vi "PH_Periodic_Sequencer.panel.vi"() -> ()   [LabVIEW 2014, in "PH_Periodic_Sequencer.lvlib"]
uses:
  PH_Periodic_Sequencer.lvlib
  PH_StatusHandler/PH_StatusHandler.GUI element.ctl
  CSCore/CSSystem/CSSystemLib/CSSystemLib.lvlib
  PH_Common/PH_Common.lvlib
  PH_Class/PH_Class.lvlib
  PH_StatusHandler/PH_StatusHandler.lvlib
panel:
  out "Delivered Shots":i32
  in  "Wanted Shots":i32
  in  "Interval [sec]":dbl=-1.0
  out "FR":T1=2 caption="State PU"
  out "MA 5":T1=2 caption="State PU"
  out "MA 4":T1=2 caption="State PU"
  out "MA 3":T1=2 caption="State PU"
  out "MA 2":T1=2 caption="State PU"
  out "MA 1":T1=2 caption="State PU"
  out "45 DP":T1=2 caption="State PU"
  out "19 DP":T1=2 caption="State PU"
  out "Seq SM State":string="no info"
  out "Ready":u32(colorbox)
  in  "Start":bool
  in  "Main Off":bool
  out "error out":errorcluster
  in  "Delete":bool
  in  "error in (no error)":errorcluster
  in  "object ref":refnum<vi>
  # "PCS"
  # "3.40"
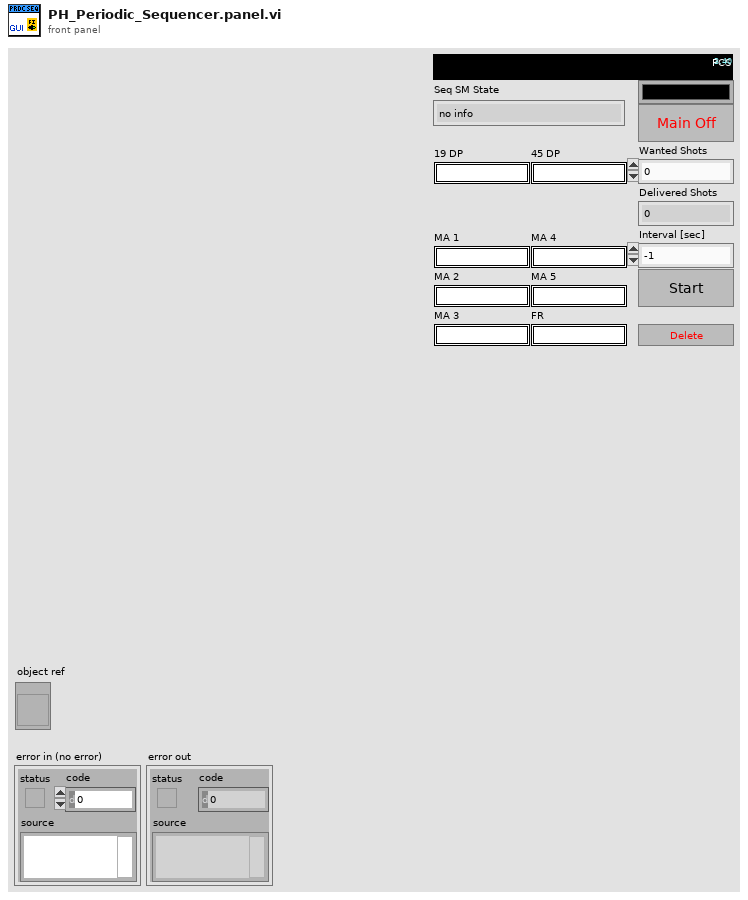
[diagram p1: front panel]
types:
  T1 = typedef "PH_StatusHandler.lvlib/PH_StatusHandler.GUI element.ctl" = u16
  T2 = typedef "PH_Periodic_Sequencer.lvlib/PH_Periodic_Sequencer.i attribute.ctl" = cluster{"GUI Refs":cluster{"Main Off":refnum<vi>, "Start":refnum<vi>, "Ready":refnum<vi>, "Sequencer SM State":refnum<vi>, "Interval [sec]":refnum<vi>, "Wanted Shots":refnum<vi>, "Delivered Shots":refnum<vi>}, "PU Info":cluster{"Instancename":string, "State":T3, "linked":bool}[], "Sequencer":cluster{"Instancename":string, "linked?":bool, "R2S?":bool, "SM State":string}, "Run?":bool, "Interval [sec]":dbl, "PU State Refs":refnum<vi>[], "Wanted Shots":i32, "Delivered Shots":i32}
  T3 = typedef "PH_StatusHandler.lvlib/PH_StatusHandler.Status.ctl" = i16
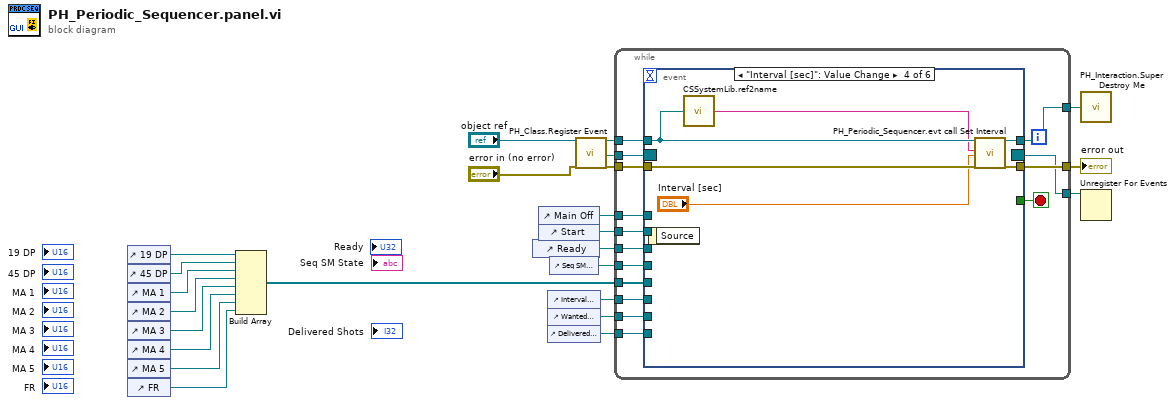
[diagram p0: block diagram]
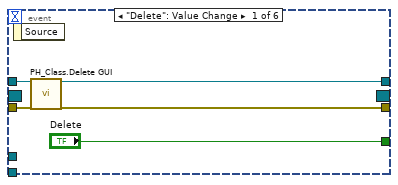
[diagram p2: hidden frame]
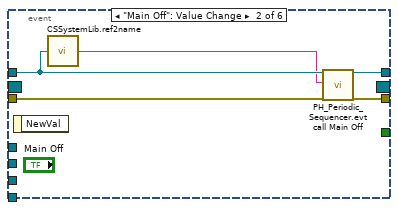
[diagram p3: hidden frame]
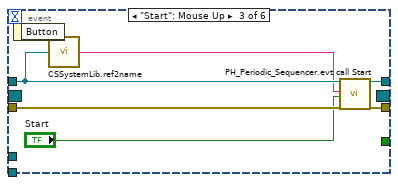
[diagram p4: hidden frame]
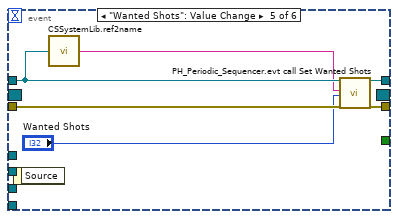
[diagram p5: hidden frame]
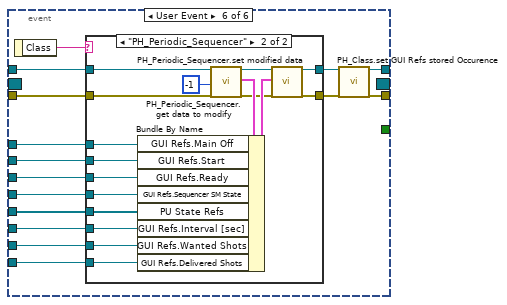
[diagram p6: hidden frame]
diagram:
  n1 = control-ref of="19 DP"() -> (w8:refnum<vi>)
  n2 = control-ref of="45 DP"() -> (w7:refnum<vi>)
  n3 = control-ref of="MA 1"() -> (w6:refnum<vi>)
  n4 = control-ref of="MA 2"() -> (w5:refnum<vi>)
  n5 = control-ref of="MA 3"() -> (w4:refnum<vi>)
  n6 = control-ref of="MA 4"() -> (w3:refnum<vi>)
  n7 = control-ref of="MA 5"() -> (w2:refnum<vi>)
  n8 = control-ref of="FR"() -> (w1:refnum<vi>)
  n9 = Build Array(w8, w7, w6, w5, w4, w3, w2, w1) -> (w14:refnum<vi>[])
  n10 = control-ref of="Ready"() -> (w16:refnum<vi>)
  n11 = control-ref of="Main Off"() -> (w18:refnum<vi>)
  n12 = control-ref of="Start"() -> (w17:refnum<vi>)
  n13 = control-ref of="Interval [sec]"() -> (w13:refnum<vi>)
  n14 = control-ref of="Wanted Shots"() -> (w12:refnum<vi>)
  n15 = control-ref of="Delivered Shots"() -> (w11:refnum<vi>)
  n16 = control-ref of="Seq SM State"() -> (w15:refnum<vi>)
  n17 = call "PH_Class.Register Event.vi"("i ref in"="object ref", "error in (no error)"="error in (no error)") -> ("i ref out"=w22:refnum<vi>, "Event Registration Refnum"=w20:refnum<event-registration>, "error out"=w21:errorcluster)  [unwired: 15 in]
  n18 = while {
    tunnel: w22 -> [w36]
    tunnel: [w35] -> w24
    tunnel: [w38] -> w23
    tunnel: w21 -> [w37]
    tunnel: w20 -> [w34]
    tunnel: [w33] -> w19
    tunnel: w18 -> [w32]
    tunnel: w17 -> [w31]
    tunnel: w16 -> [w30]
    tunnel: w15 -> [w29]
    tunnel: w14 -> [w28]
    tunnel: w13 -> [w27]
    tunnel: w12 -> [w26]
    tunnel: w11 -> [w25]
    stop <- w39 stop-if-true
    n19 = event shown="[3] \"Interval [sec]\": Value Change" {
      selector: w34 -> [_ _ _ _ _ _]
      dyn-events: [_ _ _ _ _ _] -> w33
      timeout: _ -> [_ _ _ _ _ _]
      tunnel: ["Delete" _ _ _ _ _] -> w39
      tunnel: w36 -> [w43 w47 w53 w59 w65 w80]
      tunnel: [w40 w48 w54 w60 w66 w81] -> w38
      tunnel: w37 -> [w42 w49 w55 w61 w67 w78]
      tunnel: [w41 w45 w51 w57 w63 w82] -> w35
      tunnel: w32 -> [_ _ _ _ _ w75]
      tunnel: w31 -> [_ _ _ _ _ w74]
      tunnel: w30 -> [_ _ _ _ _ w73]
      tunnel: w29 -> [_ _ _ _ _ w72]
      tunnel: w28 -> [_ _ _ _ _ w71]
      tunnel: w27 -> [_ _ _ _ _ w70]
      tunnel: w26 -> [_ _ _ _ _ w69]
      tunnel: w25 -> [_ _ _ _ _ w68]
      event "Delete": Value Change {
        n20 = event-data() -> ()  [unwired: 1 in, 1 out]
        n21 = call "PH_Class.Delete GUI.vi"("VI in"=w43, "error in (no error)"=w42) -> ("VI out"=w41:refnum<vi>, "error out"=w40:errorcluster)  [unwired: 16 in]
      }
      event "Main Off": Value Change {
        n22 = event-data() -> ()  [unwired: 1 in, 1 out]
        n23 = call "CSSystemLib.ref2name.vi"("obj refnum"=w47) -> ("name"=w46:string)
        n24 = call "PH_Periodic_Sequencer.evt call Main Off.vi"("i ref in"=w47, "Instance"=w46, "error in (no error)"=w49) -> ("i ref out"=w45:refnum<vi>, "error out"=w48:errorcluster)  [unwired: 15 in]
      }
      event "Start": Mouse Up {
        n25 = event-data() -> ()  [unwired: 1 in, 1 out]
        n26 = call "CSSystemLib.ref2name.vi"("obj refnum"=w53) -> ("name"=w52:string)
        n27 = call "PH_Periodic_Sequencer.evt call Start.vi"("i ref in"=w53, "Instance"=w52, "Start"="Start", "error in (no error)"=w55) -> ("i ref out"=w51:refnum<vi>, "error out"=w54:errorcluster)  [unwired: 14 in]
      }
      event "Interval [sec]": Value Change {
        n28 = event-data() -> ()  [unwired: 1 in, 1 out]
        n29 = call "CSSystemLib.ref2name.vi"("obj refnum"=w59) -> ("name"=w58:string)
        n30 = call "PH_Periodic_Sequencer.evt call Set Interval.vi"("i ref in"=w59, "Instance"=w58, "Interval [sec]"="Interval [sec]", "error in (no error)"=w61) -> ("i ref out"=w57:refnum<vi>, "error out"=w60:errorcluster)  [unwired: 14 in]
      }
      event "Wanted Shots": Value Change {
        n31 = event-data() -> ()  [unwired: 1 in, 1 out]
        n32 = call "CSSystemLib.ref2name.vi"("obj refnum"=w65) -> ("name"=w64:string)
        n33 = call "PH_Periodic_Sequencer.evt call Set Wanted Shots.vi"("i ref in"=w65, "Instance"=w64, "Wanted Shots"="Wanted Shots", "error in (no error)"=w67) -> ("i ref out"=w63:refnum<vi>, "error out"=w66:errorcluster)  [unwired: 14 in]
      }
      event User Event {
        n34 = event-data() -> ("Class"=w76:string)  [unwired: 1 in]
        n35 = case shown="\"PH_Periodic_Sequencer\"" w76 {
          tunnel: w80 -> [w84 w96]
          tunnel: [w84 w95] -> w79
          tunnel: w78 -> [w83 w94]
          tunnel: [w83 w93] -> w77
          tunnel: w75 -> [_ w92]
          tunnel: w74 -> [_ w91]
          tunnel: w73 -> [_ w90]
          tunnel: w72 -> [_ w89]
          tunnel: w71 -> [_ w85]
          tunnel: w70 -> [_ w88]
          tunnel: w69 -> [_ w87]
          tunnel: w68 -> [_ w86]
          frame Default {
          }
          frame "PH_Periodic_Sequencer" {
            n36 = call "PH_Periodic_Sequencer.get data to modify.vi"("i ref in"=w96, "ms timeout (10000)"=-1, "error in (no error)"=w94) -> ("i ref out"=w99:refnum<vi>, "i attribute"=w101:T2, "error out"=w97:errorcluster)  [unwired: 13 in, 1 out]
            n37 = Bundle By Name(cluster=w101, "GUI Refs.Main Off"=w92, "GUI Refs.Start"=w91, "GUI Refs.Ready"=w90, "GUI Refs.Sequencer SM State"=w89, "PU State Refs"=w85, "GUI Refs.Interval [sec]"=w88, "GUI Refs.Wanted Shots"=w87, "GUI Refs.Delivered Shots"=w86) -> (w100:T2)
            n38 = call "PH_Periodic_Sequencer.set modified data.vi"("i ref in"=w99, "i attribute"=w100, "error in (no error)"=w97) -> ("i ref out"=w95:refnum<vi>, "error out"=w93:errorcluster)  [unwired: 15 in]
          }
        }
        n39 = call "PH_Class.set GUI Refs stored Occurence.vi"("i ref in"=w79, "error in (no error)"=w77) -> ("i ref out"=w82:refnum<vi>, "error out"=w81:errorcluster)  [unwired: 16 in]
      }
    }
  }
  "error out" <- w23
  n40 = call "PH_Interaction.Super Destroy Me.vi"("i ref out"=w24) -> ()
  n41 = Unregister For Events(event registration refnum=w19) -> ()  [unwired: 1 in, 1 out]
